vi "Write_setup_to_BSA_F600.vi"(3 "No Of Samples":i32, 4 "Time (s)":sgl, 5 "BSA Setup In":T1={"Wavelength (nm)"=514.5, "Vel Comp"="W", "Max Velocity"=0.0, "Min Velocity"=0.0, "Max Record length"=2, "Signal gain (dB)"=30, "High voltage"=2000, "Optics Conversion Factor"=0.0, "Min Record length"=2, "Multiply Velocity by -1"=FALSE, "Signal to Noise Ratio"="0", "Validation Ratio"="4", "Probe"="", "Laser"="", "BSA"="", "Lense"="", "Beam Separation (mm)"=514.5, "Focal Length (mm)"=514.5, "COLOUR"=52224, "BSA IP"="", "Velocity Range (m/s)"=0.0, "Centre Velocity (m/s)"=0.0, "Unshifted mW"=0.0, "Shifted mW"=0.0, "Bandwidth Hz"=0.0, "Req Sampling Rate Hz"=100.0, "Ch"=0, "CenterFreq Hz"=0.0, "Laser IP"=""} {"Req Sampling Rate Hz" min=1.0; "Shifted mW" format="%.1g"; "Unshifted mW" format="%.1g"; "Centre Velocity (m/s)" format="%.2g"; "Velocity Range (m/s)" format="%.2g"; "Focal Length (mm)" format="%.1f"; "Beam Separation (mm)" format="%.1f"; "Optics Conversion Factor" format="%.3g"; "High voltage" min=0 max=2040 step=8; "Signal gain (dB)" min=0 max=30 step=1; "Min Velocity" format="%.2g"; "Max Velocity" format="%.2g"; "Wavelength (nm)" format="%.1f"}, 6 "BSACtrl.IBSA F600":refnum<k7>) -> (0 "error out":errorcluster, 1 "Frequecy Shift (MHz)":i32, 2 "BSACtrl.IBSA F600 Out":refnum<k7>)   [LabVIEW 2020]
uses:
  LDA_Channel.ctl
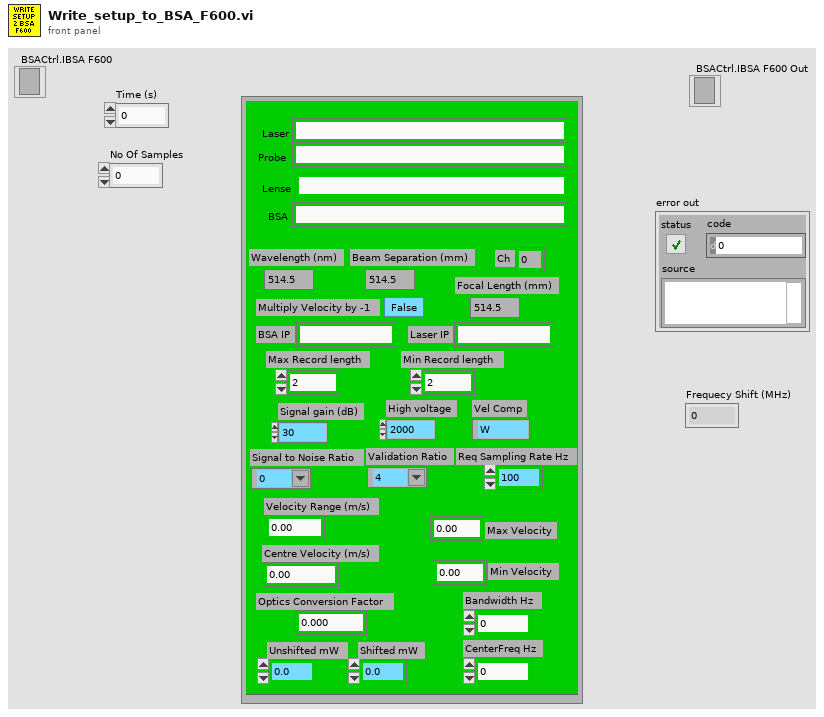
[diagram p1: front panel]
types:
  T1 = typedef "LDA_Channel.ctl" = cluster{"Wavelength (nm)":dbl, "Vel Comp":string, "Max Velocity":dbl, "Min Velocity":dbl, "Max Record length":u16, "Signal gain (dB)":i16, "High voltage":i16, "Optics Conversion Factor":dbl, "Min Record length":u16, "Multiply Velocity by -1":bool, "Signal to Noise Ratio":string, "Validation Ratio":string, "Probe":string, "Laser":string, "BSA":string, "Lense":string, "Beam Separation (mm)":dbl, "Focal Length (mm)":dbl, "COLOUR":u32, "BSA IP":string, "Velocity Range (m/s)":dbl, "Centre Velocity (m/s)":dbl, "Unshifted mW":dbl, "Shifted mW":dbl, "Bandwidth Hz":dbl, "Req Sampling Rate Hz":dbl, "Ch":i32, "CenterFreq Hz":dbl, "Laser IP":string}
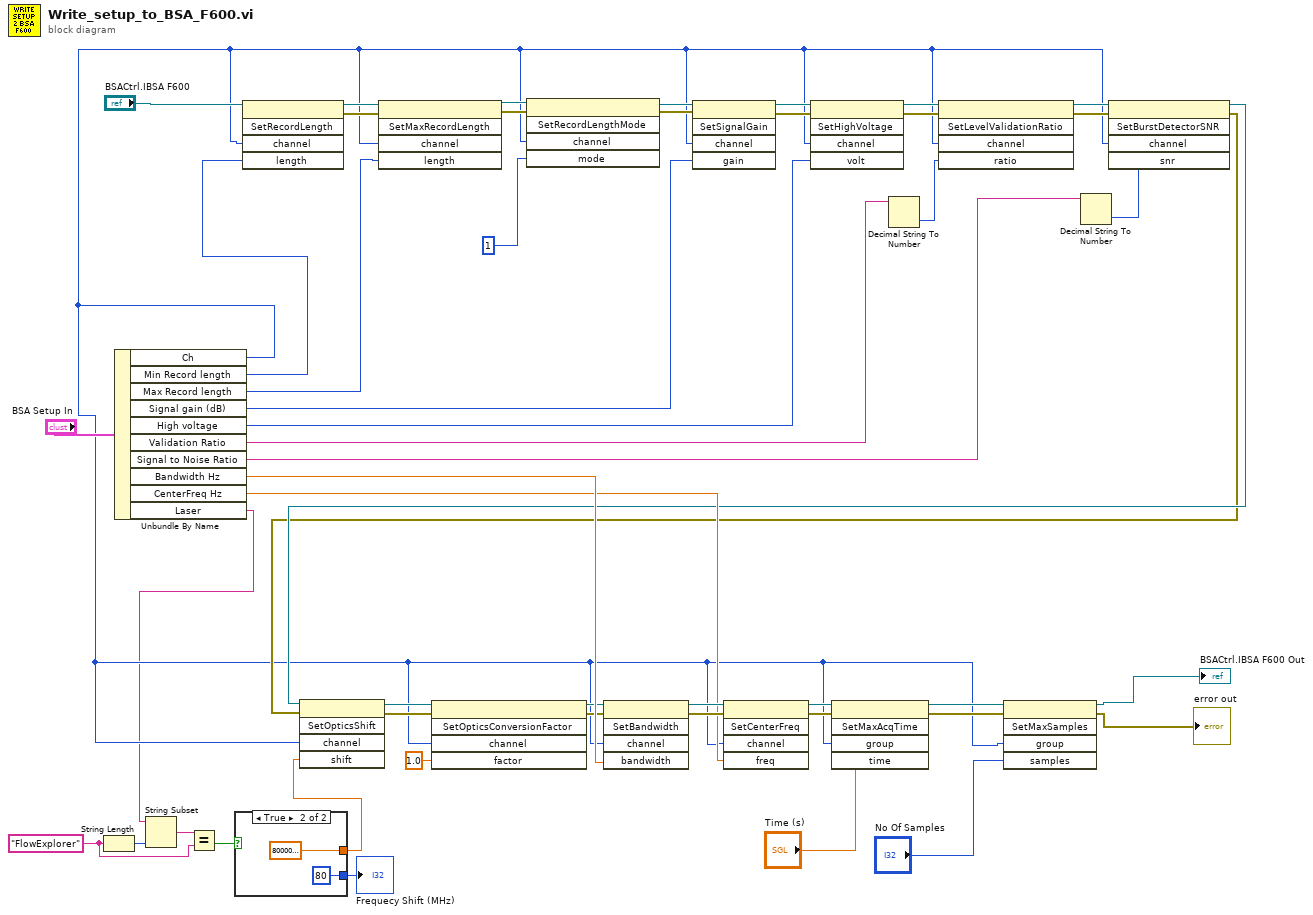
[diagram p0: block diagram]
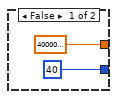
[diagram p2: hidden frame]
diagram:
  w4 = "FlowExplorer"
  n1 = String Length(string=w4) -> (length=w7:i32)
  n2 = Unbundle By Name("BSA Setup In") -> ("Ch"=w10:i32, "Min Record length"=w20:u16, "Max Record length"=w19:u16, "Signal gain (dB)"=w34:i16, "High voltage"=w33:i16, "Validation Ratio"=w32:string, "Signal to Noise Ratio"=w29:string, "Bandwidth Hz"=w28:dbl, "CenterFreq Hz"=w27:dbl, "Laser"=w6:string)
  n3 = String Subset(string=w6, length (rest)=w7) -> (substring=w5:string)  [unwired: 1 in]
  n4 = Equal?(x=w5, y=w4) -> (x = y?=w3:bool)
  n5 = case shown="True" w3 {
    tunnel: [sgl 40000000.0 ("shift") sgl 80000000.0 ("shift")] -> w2
    tunnel: [40 ("shift") 80 ("shift")] -> w1
    frame False {
    }
    frame True {
    }
  }
  "Frequecy Shift (MHz)" <- w1
  n6 = invoke method="SetRecordLength"(reference="BSACtrl.IBSA F600", "channel"=w10, "length"=w20) -> (reference out=w49:refnum<k7>, error out=w40:errorcluster)  [unwired: 2 in, 3 out]
  n7 = invoke method="SetMaxRecordLength"(reference=w49, error in=w40, "channel"=w10, "length"=w19) -> (reference out=w39:refnum<k7>, error out=w38:errorcluster)  [unwired: 1 in, 3 out]
  n8 = invoke method="SetRecordLengthMode"(reference=w39, error in=w38, "channel"=w10, "mode"=1) -> (reference out=w37:refnum<k7>, error out=w36:errorcluster)  [unwired: 1 in, 3 out]
  n9 = invoke method="SetSignalGain"(reference=w37, error in=w36, "channel"=w10, "gain"=w34) -> (reference out=w48:refnum<k7>, error out=w41:errorcluster)  [unwired: 1 in, 3 out]
  n10 = invoke method="SetHighVoltage"(reference=w48, error in=w41, "channel"=w10, "volt"=w33) -> (reference out=w47:refnum<k7>, error out=w42:errorcluster)  [unwired: 1 in, 3 out]
  n11 = Decimal String To Number(string=w32) -> (number=w31:i32)  [unwired: 3 out]
  n12 = invoke method="SetLevelValidationRatio"(reference=w47, error in=w42, "channel"=w10, "ratio"=w31) -> (reference out=w46:refnum<k7>, error out=w43:errorcluster)  [unwired: 1 in, 3 out]
  n13 = Decimal String To Number(string=w29) -> (number=w30:i32)  [unwired: 3 out]
  n14 = invoke method="SetBurstDetectorSNR"(reference=w46, error in=w43, "channel"=w10, "snr"=w30) -> (reference out=w14:refnum<k7>, error out=w13:errorcluster)  [unwired: 1 in, 3 out]
  n15 = invoke method="SetOpticsShift"(reference=w14, error in=w13, "channel"=w10, "shift"=w2) -> (reference out=w17:refnum<k7>, error out=w16:errorcluster)  [unwired: 1 in, 3 out]
  n16 = invoke method="SetOpticsConversionFactor"(reference=w17, error in=w16, "channel"=w10, "factor"=sgl 1.0) -> (reference out=w12:refnum<k7>, error out=w11:errorcluster)  [unwired: 1 in, 3 out]
  n17 = invoke method="SetBandwidth"(reference=w12, error in=w11, "channel"=w10, "bandwidth"=w28) -> (reference out=w45:refnum<k7>, error out=w44:errorcluster)  [unwired: 1 in, 3 out]
  n18 = invoke method="SetCenterFreq"(reference=w45, error in=w44, "channel"=w10, "freq"=w27) -> (reference out=w24:refnum<k7>, error out=w23:errorcluster)  [unwired: 1 in, 3 out]
  n19 = invoke method="SetMaxAcqTime"(reference=w24, error in=w23, "group"=w10, "time"="Time (s)") -> (reference out=w25:refnum<k7>, error out=w26:errorcluster)  [unwired: 1 in, 3 out]
  n20 = invoke method="SetMaxSamples"(reference=w25, error in=w26, "group"=w10, "samples"="No Of Samples") -> (reference out=→"BSACtrl.IBSA F600 Out":refnum<k7>, error out=→"error out":errorcluster)  [unwired: 1 in, 3 out]
